vi "eFinanceN.vi"(11 "file path":path) -> (0 "double precision float":dbl format="%#_8g", 1 "Tabel as Arr":string[](array[string]), 2 "Cash as DBL":dbl[](array[numeric]), 3 "Concatenated String":string)   [LabVIEW 2023]
uses:
  <vilib>/Utility/file.llb/Read Delimited Spreadsheet (string).vi
panel:
  out "Cash as Str":string[](array[string])
  in  "default (0 I32)":u32
  out "before 2 sub":string
  out "before 1 sub":string
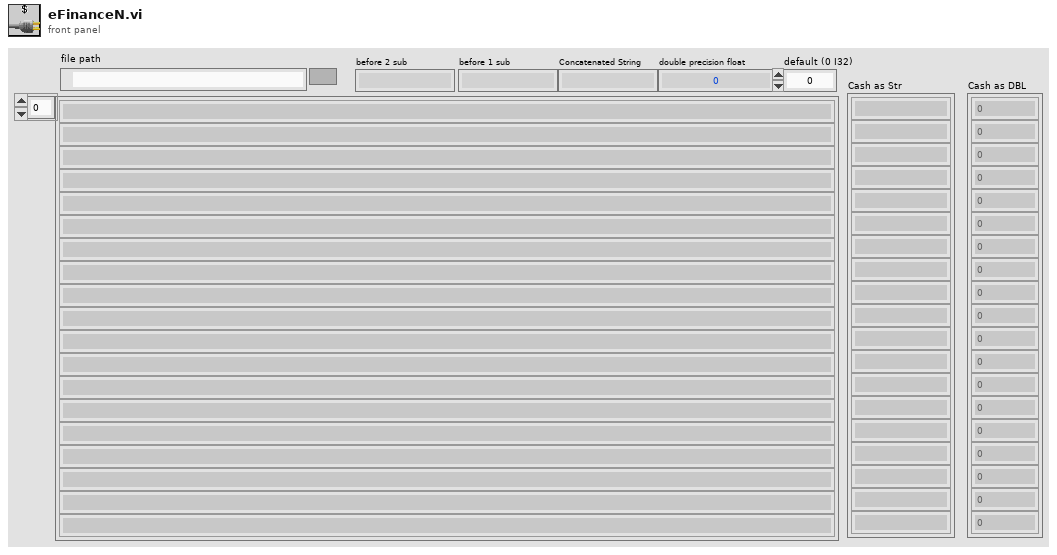
[diagram p1: front panel]
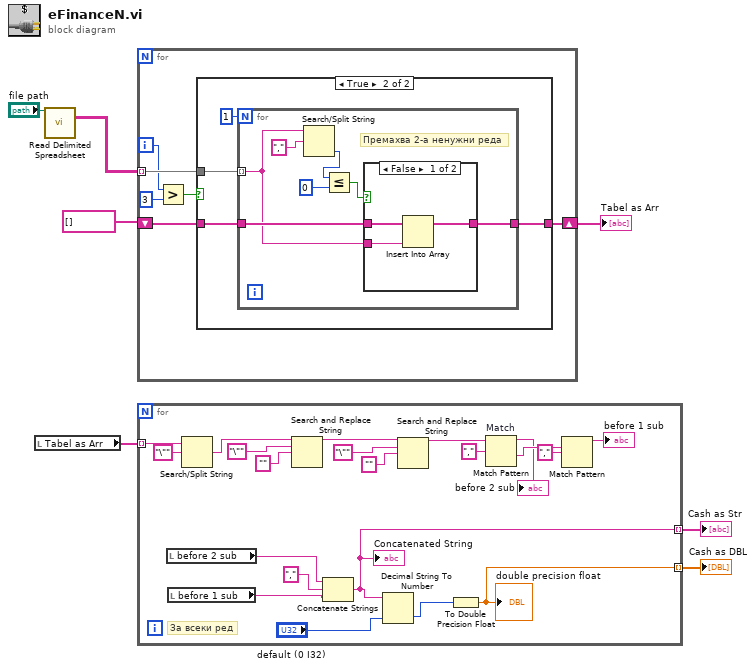
[diagram p0: block diagram]
diagram:
  n1 = local read "Tabel as Arr"() -> (w3:string[])
  n2 = call-poly <vilib>:"Read Delimited Spreadsheet.vi"("file path (dialog if empty)"="file path") -> ("all rows"=w4:string[][])  [unwired: 9 in, 5 out]
  n3 = for {
    tunnel: w4 -> [w13] mode=indexing
    shift-right: [w12] -> w5
    shift-left: string[] [] -> [w11]
    i -> [w8]
    n4 = Greater?(x=w8, y=3) -> (0:w10:bool)
    n5 = case shown="True" w10 {
      tunnel: w13 -> [_ w18]
      tunnel: [w14 w16] -> w12
      tunnel: w11 -> [w14 w15]
      frame False {
      }
      frame True {
        n6 = for {
          N: 1 -> [_]
          tunnel: w18 -> [w20] mode=indexing
          tunnel: [w25] -> w16
          tunnel: w15 -> [w24]
          # "Премахва 2-а ненужни реда"
          n7 = Search/Split String(string=w20, search string/char (-)="," ("regular expression")) -> (offset of match=w19:i32)  [unwired: 1 in, 2 out]
          n8 = Less Or Equal?(x=w19, y=0) -> (x <= y?=w23:bool)
          n9 = case shown="False" w23 {
            tunnel: w20 -> [w28 _]
            tunnel: [w27 w29] -> w25
            tunnel: w24 -> [w26 w29]
            frame False {
              n10 = Insert Into Array(array=w26, new element=w28) -> (w27:string[])  [unwired: 1 in]
            }
            frame True {
            }
          }
        }
      }
    }
  }
  "Tabel as Arr" <- w5
  n11 = for {
    tunnel: w3 -> [w50] mode=indexing
    tunnel: [w33] -> w2 mode=indexing
    tunnel: [w30] -> w1 mode=indexing
    # "За всеки ред"
    n12 = local read "before 2 sub"() -> (w34:string)
    n13 = local read "before 1 sub"() -> (w36:string)
    n14 = Search/Split String(string=w50, search string/char (-)="\"") -> (match + rest of string=w48:string)  [unwired: 1 in, 2 out]
    n15 = Search and Replace String(input string=w48, search string="\"", replace string="" ("replace string (\"\")")) -> (result string=w43:string)  [unwired: 5 in, 3 out]
    n16 = Concatenate Strings "Concatenate Strings"(w34, ",", w36) -> (w33:string)
    "Concatenated String" <- w33
    n17 = Decimal String To Number(string=w33, default (0L)="default (0 I32)") -> (number=w32:u32)  [unwired: 1 in, 1 out]
    n18 = Search and Replace String(input string=w43, search string="\"", replace string="" ("replace string (\"\")")) -> (result string=w38:string)  [unwired: 5 in, 3 out]
    n19 = To Double Precision Float(number=w32) -> (double precision float=w30:dbl)
    "double precision float" <- w30
    n20 = Match Pattern "Match"(string=w38, regular expression=",") -> (before substring=→"before 2 sub":string, after substring=w40:string)  [unwired: 1 in, 2 out]
    n21 = Match Pattern(string=w40, regular expression=",") -> (before substring=→"before 1 sub":string)  [unwired: 1 in, 3 out]
  }
  "Cash as Str" <- w2
  "Cash as DBL" <- w1
